vi "Wait Update.vi"(0 "VISA resource name":refnum<visa-resource-name>, 11 "error in (no error)":errorcluster) -> (4 "VISA resource name out":refnum<visa-resource-name>, 15 "error out":errorcluster)   [LabVIEW 2013, in "Yokogawa.lvlib" / "Yokogawa PZ4000.lvlib"]
doc: "This VI waits to finished the Updating for the PZ4000 series.\nWait complited to Start and Stop.\nUpdate Functions are clear Status, Set Filter, Set Extended Event Status Enable Register, Get Extended Event Status Register, Send Start, Wait Extended Event(start complited), clear Status, Set Filter, Set Extended Event Status Enable Register, Get Extended Event Status Register, Send Stop, Wait Extended Event(stop complited)."
uses:
  Yokogawa PZ4000.lvlib
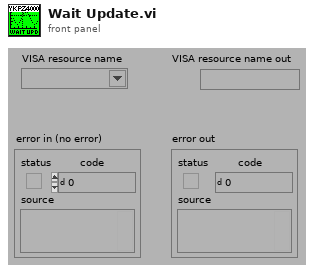
[diagram p1: front panel]
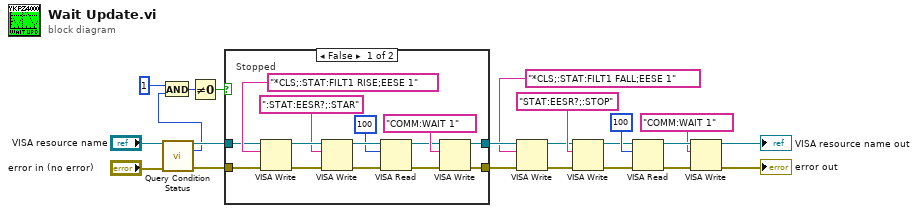
[diagram p0: block diagram]
diagram:
  n1 = call "Query Condition Status.vi"("VISA resource name"="VISA resource name", "error in (no error)"="error in (no error)") -> ("VISA resource name out"=w9:refnum<visa-resource-name>, "Condition"=w1:i32, "error out"=w10:errorcluster)  [unwired: 11 in]
  n2 = And(x=1, y=w1) -> (x .and. y?=w7:i32)
  n3 = Not Equal To 0?(x=w7) -> (x != 0?=w8:bool)
  n4 = case shown="False" w8 {
    tunnel: [w36 w38] -> w14
    tunnel: [w35 w37] -> w15
    tunnel: w10 -> [w31 w37]
    tunnel: w9 -> [w30 w38]
    frame False {
      # "Stopped"
      n5 = VISA Write(VISA resource name=w30, write buffer="*CLS;:STAT:FILT1 RISE;EESE 1", error in (no error)=w31) -> (VISA resource name out=w33:refnum<visa-resource-name>, error out=w32:errorcluster)  [unwired: 1 out]
      n6 = VISA Write(VISA resource name=w33, write buffer=":STAT:EESR?;:STAR", error in (no error)=w32) -> (VISA resource name out=w28:refnum<visa-resource-name>, error out=w29:errorcluster)  [unwired: 1 out]
      n7 = VISA Read(VISA resource name=w28, byte count=100, error in (no error)=w29) -> (VISA resource name out=w26:refnum<visa-resource-name>, error out=w25:errorcluster)  [unwired: 2 out]
      n8 = VISA Write(VISA resource name=w26, write buffer="COMM:WAIT 1", error in (no error)=w25) -> (VISA resource name out=w36:refnum<visa-resource-name>, error out=w35:errorcluster)  [unwired: 1 out]
    }
    frame True {
      # "Running"
    }
  }
  n9 = VISA Write(VISA resource name=w14, write buffer="*CLS;:STAT:FILT1 FALL;EESE 1", error in (no error)=w15) -> (VISA resource name out=w13:refnum<visa-resource-name>, error out=w12:errorcluster)  [unwired: 1 out]
  n10 = VISA Write(VISA resource name=w13, write buffer="STAT:EESR?;:STOP", error in (no error)=w12) -> (VISA resource name out=w17:refnum<visa-resource-name>, error out=w16:errorcluster)  [unwired: 1 out]
  n11 = VISA Read(VISA resource name=w17, byte count=100, error in (no error)=w16) -> (VISA resource name out=w19:refnum<visa-resource-name>, error out=w20:errorcluster)  [unwired: 2 out]
  n12 = VISA Write(VISA resource name=w19, write buffer="COMM:WAIT 1", error in (no error)=w20) -> (VISA resource name out=→"VISA resource name out":refnum<visa-resource-name>, error out=→"error out":errorcluster)  [unwired: 1 out]
